vi "MyCircBuffTest.vi"() -> ()   [LabVIEW 2013]
uses:
  My circular buffer info.ctl
panel:
  in  "stop":bool
  in  "Event Click":bool
  out "Waveform Graph":i16[][](graph)
  out "write pointer (block position)":i32
  in  "buffer2 path":path
  in  "buffer1 path":path
  in  "archive directory":path
  in  "num blocks  prior":i32
  in  "num blocks after":i32
  in  "bytes/sample":i32
  in  "samples/block/channel":i32
  in  "number of channels":i32
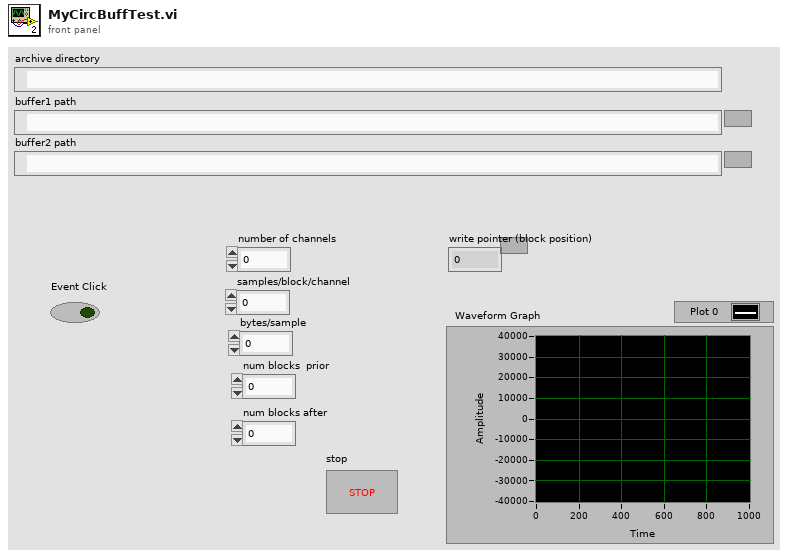
[diagram p1: front panel]
types:
  T1 = typedef "My circular buffer info.ctl" = cluster{"buff ref1":refnum<file>, "buff ref2":refnum<file>, "buffer1 path":path, "buffer2 path":path, "archive directory":path, "xml header":string, "num blocks  prior":i32, "num blocks after":i32, "blocks/event":i32, "samples/block":i32, "bytes/sample":i32, "number of channels":i32, "samples/block/channel":i32, "read buffer ref queue":refnum<queue>, "Event delay queue":refnum<queue>, "command queue":refnum<queue>}
  T2 = cluster{"filename":string, "bytes to write":i32, "archive mode":enum16{"direct", "append"}}
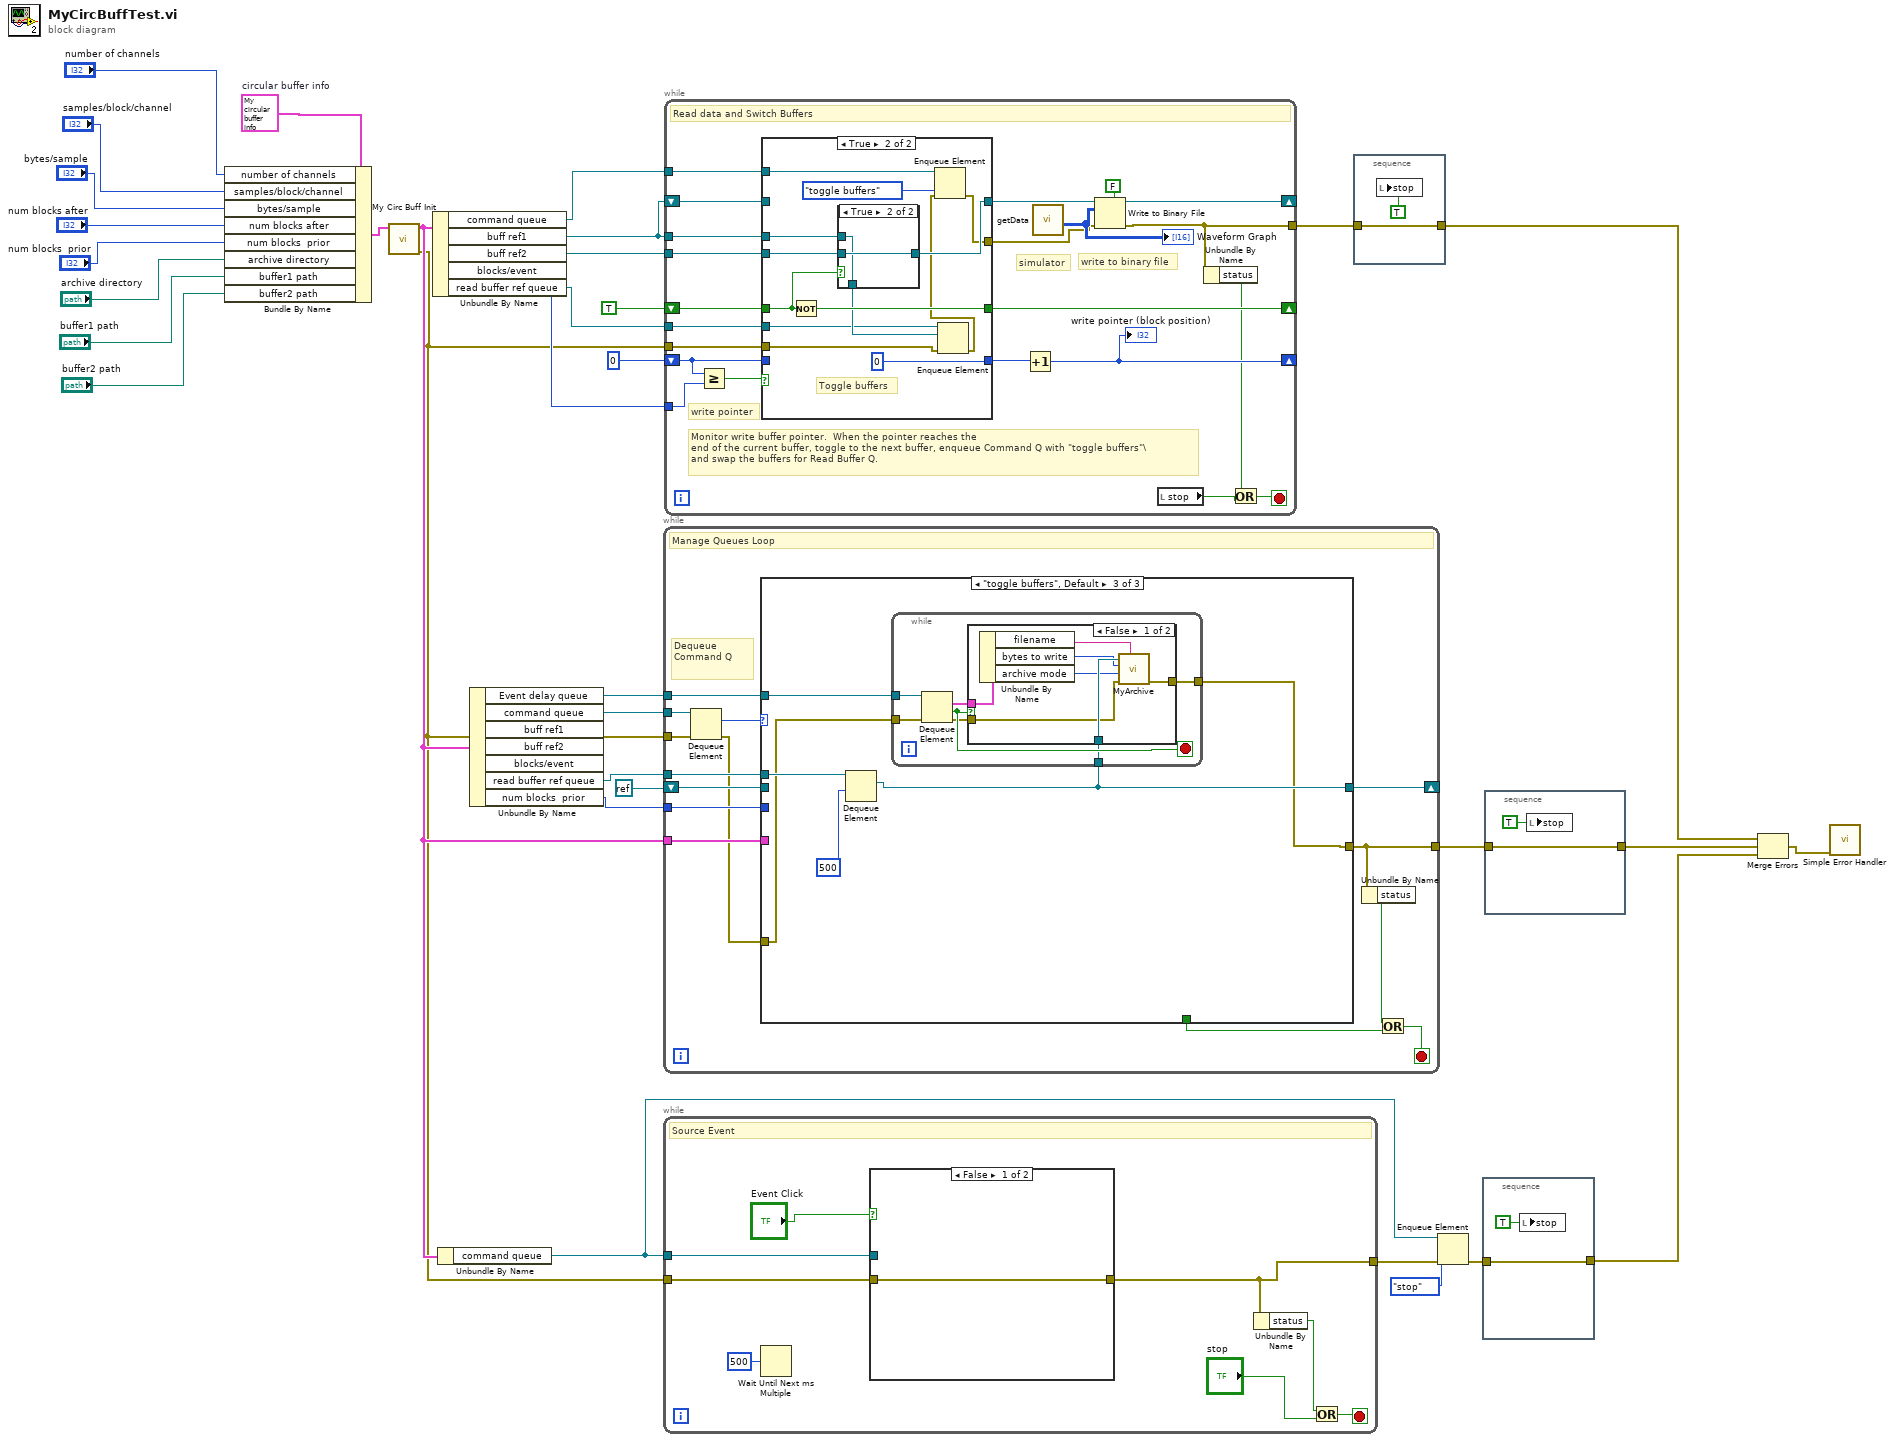
[diagram p0: block diagram]
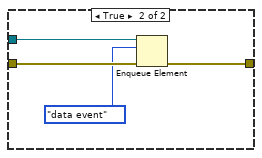
[diagram p2: hidden frame]
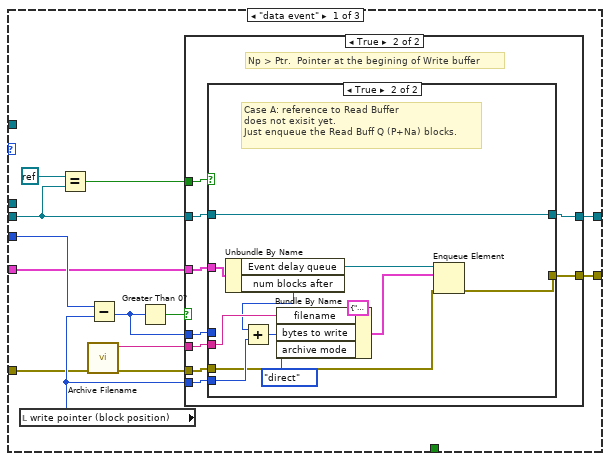
[diagram p3: hidden frame]
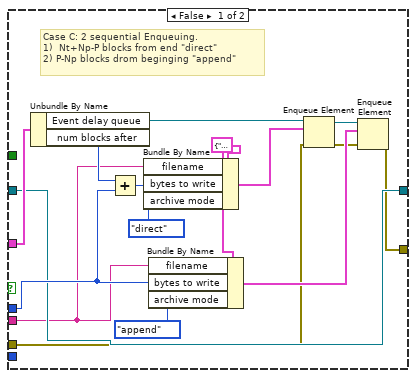
[diagram p4: hidden frame]
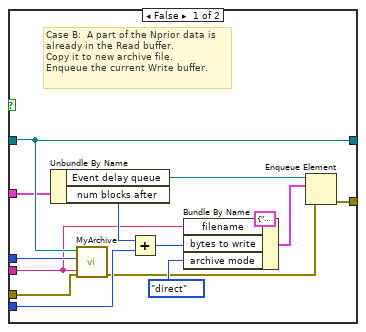
[diagram p5: hidden frame]
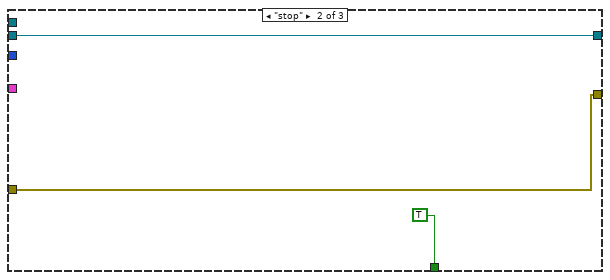
[diagram p6: hidden frame]
diagram:
  w29 = T1 {"buff ref1"=refnum, "buff ref2"=refnum, "buffer1 path"=path "", "buffer2 path"=path "", "archive directory"=path "", "xml header"="", "num blocks  prior"=0, "num blocks after"=0, "blocks/event"=0, "samples/block"=0, "bytes/sample"=0, "number of channels"=0, "samples/block/channel"=0, "read buffer ref queue"=refnum, "Event delay queue"=refnum, "command queue"=refnum}  # circular buffer info
  n1 = Bundle By Name(cluster=w29, "number of channels"="number of channels", "samples/block/channel"="samples/block/channel", "bytes/sample"="bytes/sample", "num blocks after"="num blocks after", "num blocks  prior"="num blocks  prior", "archive directory"="archive directory", "buffer1 path"="buffer1 path", "buffer2 path"="buffer2 path") -> (w25:T1)
  n2 = call "My Circ Buff Init.vi"("circular buffer info"=w25) -> ("error out"=w6:errorcluster, "circular buffer info out"=w12:T1)  [unwired: 9 in]
  n3 = Unbundle By Name(w12) -> ("command queue"=w18:refnum<queue>, "buff ref1"=w20:refnum<file>, "buff ref2"=w22:refnum<file>, "blocks/event"=w24:i32, "read buffer ref queue"=w19:refnum<queue>)
  n4 = Unbundle By Name(w12) -> ("command queue"=w11:refnum<queue>)
  n5 = Unbundle By Name(w12) -> ("Event delay queue"=w13:refnum<queue>, "command queue"=w17:refnum<queue>, "read buffer ref queue"=w14:refnum<queue>, "num blocks  prior"=w15:i32)  [unwired: 3 out]
  n6 = while {
    tunnel: w17 -> [w48]
    shift-right: [w44] -> _
    shift-left: refnum<k0> refnum -> [w47]
    tunnel: w15 -> [w46]
    tunnel: w12 -> [w45]
    tunnel: w14 -> [w43]
    tunnel: w13 -> [w42]
    tunnel: w6 -> [w41]
    tunnel: [w39] -> w7
    stop <- w36 stop-if-true
    # "Dequeue \nCommand Q"
    # "Manage Queues Loop"
    n7 = Dequeue Element(queue=w48, error in (no error)=w41) -> (element=w35:enum16{"toggle buffers", "data event", "stop"}, error out=w40:errorcluster)  [unwired: 1 in, 2 out]
    n8 = case shown="\"toggle buffers\", Default" w35 {
      tunnel: w47 -> [w55 w115 _]
      tunnel: w46 -> [w59 _ _]
      tunnel: w45 -> [w57 _ _]
      tunnel: [w54 w115 w119] -> w44
      tunnel: w43 -> [_ _ w121]
      tunnel: w42 -> [_ _ w120]
      tunnel: [_ TRUE _] -> w37
      tunnel: w40 -> [w51 w113 w117]
      tunnel: [w49 w113 w116] -> w39
      frame "data event" {
        n9 = local read "write pointer (block position)"() -> (w52:i32)
        n10 = Equal?(x=refnum<k0> refnum, y=w55) -> (x = y?=w60:bool)
        n11 = call "Archive Filename.vi"("error in (no error)"=w51) -> ("error out"=w50:errorcluster, "filename"=w53:string)  [unwired: 9 in]
        n12 = Subtract(x=w59, y=w52) -> (x-y=w56:i32)
        n13 = Greater Than 0?(x=w56) -> (x > 0?=w58:bool)
        n14 = case shown="True" w58 {
          tunnel: w60 -> [_ w86]
          tunnel: w57 -> [w67 w85]
          tunnel: w56 -> [w70 w84]
          tunnel: w55 -> [w66 w83]
          tunnel: [w66 w82] -> w54
          tunnel: w53 -> [w65 w81]
          tunnel: w52 -> [_ w80]
          tunnel: w50 -> [w64 w79]
          tunnel: [w62 w78] -> w49
          frame False {
            w69 = T2 {"filename"="", "bytes to write"=0, "archive mode"=enum."direct"} ("Event delay info")
            # "Case C: 2 sequential Enqueuing. \n1)  Nt+Np-P blocks from end \"direct\"\n2) P-Np blocks drom beginging \"append\""
            n15 = Unbundle By Name(w67) -> ("Event delay queue"=w77:refnum<queue>, "num blocks after"=w73:i32)
            n16 = Add(x=w73, y=w70) -> (x+y=w74:i32)
            n17 = Bundle By Name(cluster=w69, "filename"=w65, "bytes to write"=w74, "archive mode"=enum16{"direct", "append"}."direct") -> (w75:T2)
            n18 = Bundle By Name(cluster=w69, "filename"=w65, "bytes to write"=w70, "archive mode"=enum16{"direct", "append"}."append") -> (w68:T2)
            n19 = Enqueue Element(queue=w77, element=w75, error in (no error)=w64) -> (queue out=w72:refnum<queue>, error out=w63:errorcluster)  [unwired: 1 in, 1 out]
            n20 = Enqueue Element(queue=w72, element=w68, error in (no error)=w63) -> (error out=w62:errorcluster)  [unwired: 1 in, 2 out]
          }
          frame True {
            # "Np > Ptr.  Pointer at the begining of Write buffer"
            n21 = case shown="True" w86 {
              tunnel: w85 -> [w93 w112]
              tunnel: w84 -> [w100 _]
              tunnel: w83 -> [w99 w107]
              tunnel: [w99 w107] -> w82
              tunnel: w81 -> [w90 w106]
              tunnel: w80 -> [w92 w103]
              tunnel: w79 -> [w89 w102]
              tunnel: [w87 w101] -> w78
              frame False {
                # "Case B:  A part of the Nprior data is\nalready in the Read buffer.  \nCopy it to new archive file.\nEnqueue the current Write buffer."
                n22 = Unbundle By Name(w93) -> ("Event delay queue"=w98:refnum<queue>, "num blocks after"=w91:i32)
                n23 = call "MyArchive.vi"("archive filename"=w90, "error in"=w89, "blocks to write"=w100, "ReadBuff refnum"=w99) -> ("error out"=w88:errorcluster)  [unwired: 5 in]
                n24 = Add(x=w91, y=w92) -> (x+y=w94:i32)
                n25 = Bundle By Name(cluster=T2 {"filename"="", "bytes to write"=0, "archive mode"=enum."direct"} ("Event delay info"), "filename"=w90, "bytes to write"=w94, "archive mode"=enum16{"direct", "append"}."direct") -> (w95:T2)
                n26 = Enqueue Element(queue=w98, element=w95, error in (no error)=w88) -> (error out=w87:errorcluster)  [unwired: 1 in, 2 out]
              }
              frame True {
                # "Case A: reference to Read Buffer \ndoes not exisit yet. \nJust enqueue the Read Buff Q (P+Na) blocks."
                n27 = Unbundle By Name(w112) -> ("Event delay queue"=w111:refnum<queue>, "num blocks after"=w104:i32)
                n28 = Add(x=w104, y=w103) -> (x+y=w105:i32)
                n29 = Bundle By Name(cluster=T2 {"filename"="", "bytes to write"=0, "archive mode"=enum."direct"} ("Event delay info"), "filename"=w106, "bytes to write"=w105, "archive mode"=enum16{"direct", "append"}."direct") -> (w108:T2)
                n30 = Enqueue Element(queue=w111, element=w108, error in (no error)=w102) -> (error out=w101:errorcluster)  [unwired: 1 in, 2 out]
              }
            }
          }
        }
      }
      frame "stop" {
      }
      frame "toggle buffers", Default {
        n31 = Dequeue Element(queue=w121, timeout in ms (-1)=500) -> (element=w119:refnum<file>)  [unwired: 1 in, 3 out]
        n32 = while {
          tunnel: w120 -> [w128]
          tunnel: w119 -> [w126]
          tunnel: w117 -> [w124]
          tunnel: [w122] -> w116
          stop <- w127 stop-if-true
          n33 = Dequeue Element(queue=w128, error in (no error)=w124) -> (element=w125:T2, timed out?=w127:bool, error out=w123:errorcluster)  [unwired: 1 in, 1 out]
          n34 = case shown="False" w127 {
            tunnel: w126 -> [w135 _]
            tunnel: w125 -> [w134 _]
            tunnel: w123 -> [w130 w136]
            tunnel: [w129 w136] -> w122
            frame False {
              n35 = Unbundle By Name(w134) -> ("filename"=w131:string, "bytes to write"=w132:i32, "archive mode"=w133:enum16{"direct", "append"})
              n36 = call "MyArchive.vi"("archive filename"=w131, "error in"=w130, "archive mode"=w133, "blocks to write"=w132, "ReadBuff refnum"=w135) -> ("error out"=w129:errorcluster)  [unwired: 4 in]
            }
            frame True {
              # "no event waits"
            }
          }
        }
      }
    }
    n37 = Unbundle By Name(w39) -> ("status"=w38:bool)
    n38 = Or(x=w38, y=w37) -> (x .or. y?=w36:bool)
  }
  n39 = while {
    tunnel: w11 -> [w144]
    tunnel: w6 -> [w143]
    tunnel: [w141] -> w5
    stop <- w142 stop-if-true
    # "Source Event"
    n40 = Wait Until Next ms Multiple(millisecond multiple=u32 500) -> ()  [unwired: 1 out]
    n41 = case shown="False" "Event Click" {
      tunnel: w144 -> [_ w149]
      tunnel: w143 -> [w145 w148]
      tunnel: [w145 w147] -> w141
      frame False {
      }
      frame True {
        n42 = Enqueue Element(queue=w149, element=enum16{"data event", "toggle buffers", "stop"}."data event", error in (no error)=w148) -> (error out=w147:errorcluster)  [unwired: 1 in, 2 out]
      }
    }
    n43 = Unbundle By Name(w141) -> ("status"=w140:bool)
    n44 = Or(x=w140, y="stop") -> (x .or. y?=w142:bool)
  }
  n45 = while {
    tunnel: w24 -> [w170]
    shift-right: [w166] -> _
    shift-left: 0 -> [w168]
    shift-right: [w163] -> _
    shift-left: w20 -> [w164]
    tunnel: w22 -> [w162]
    shift-right: [w160] -> _
    shift-left: TRUE -> [w161]
    tunnel: w20 -> [w159]
    tunnel: w19 -> [w158]
    tunnel: w18 -> [w157]
    tunnel: w6 -> [w155]
    tunnel: [w151] -> w8
    stop <- w153 stop-if-true
    # "Monitor write buffer pointer.  When the pointer reaches the \nend of the current buffer, toggle to the next buffer, enqueue Command Q with \"toggle buffers\"\\\nand swap the buffers for Read Buffer Q."
    # "write pointer"
    # "simulator"
    # "write to binary file"
    # "Read data and Switch Buffers"
    n46 = Greater Or Equal?(x=w168, y=w170) -> (x >= y?=w169:bool)
    n47 = case shown="True" w169 {
      tunnel: w168 -> [w175 _]
      tunnel: [w175 0] -> w167
      tunnel: [w174 w185] -> w165
      tunnel: w164 -> [w174 _]
      tunnel: w162 -> [_ w186]
      tunnel: w161 -> [w173 w187]
      tunnel: [w173 w188] -> w160
      tunnel: w159 -> [_ w184]
      tunnel: w158 -> [_ w182]
      tunnel: w157 -> [_ w181]
      tunnel: w155 -> [w172 w179]
      tunnel: [w172 w177] -> w154
      frame False {
      }
      frame True {
        # "Toggle buffers"
        n48 = Not(x=w187) -> (.not. x?=w188:bool)
        n49 = case shown="True" w187 {
          tunnel: w186 -> [w189 w192]
          tunnel: [w190 w192] -> w185
          tunnel: w184 -> [w190 w191]
          tunnel: [w189 w191] -> w183
          frame False {
          }
          frame True {
          }
        }
        n50 = Enqueue Element(queue=w182, element=w183, error in (no error)=w179) -> (error out=w178:errorcluster)  [unwired: 1 in, 2 out]
        n51 = Enqueue Element(queue=w181, element=enum16{"toggle buffers", "data event", "stop"}."toggle buffers", error in (no error)=w178) -> (error out=w177:errorcluster)  [unwired: 1 in, 2 out]
      }
    }
    n52 = Increment(x=w167) -> (x+1=w166:i32)
    "write pointer (block position)" <- w166
    n53 = call "getData.vi"() -> ("binary data"=w156:i16[][])  [unwired: 7 in]
    "Waveform Graph" <- w156
    n54 = Write to Binary File(file (use dialog)=w165, data=w156, error in=w154, 5:FALSE ("prepend array or string size? (T)")) -> (refnum out=w163:refnum<file>, error out=w151:errorcluster)  [unwired: 2 in, 1 out]
    n55 = local read "stop"() -> (w152:bool)
    n56 = Unbundle By Name(w151) -> ("status"=w150:bool)
    n57 = Or(x=w150, y=w152) -> (x .or. y?=w153:bool)
  }
  n58 = stacked-sequence {
    tunnel: w8 -> [w194]
    tunnel: [w194] -> w4
    frame #0 {
      n59 = local write "stop"(TRUE ("stop")) -> ()
    }
  }
  n60 = Enqueue Element(queue=w11, element=enum16{"data event", "toggle buffers", "stop"}."stop", error in (no error)=w5) -> (error out=w9:errorcluster)  [unwired: 1 in, 2 out]
  n61 = stacked-sequence {
    tunnel: w9 -> [w196]
    tunnel: [w196] -> w2
    frame #0 {
      n62 = local write "stop"(TRUE ("stop")) -> ()
    }
  }
  n63 = stacked-sequence {
    tunnel: w7 -> [w198]
    tunnel: [w198] -> w3
    frame #0 {
      n64 = local write "stop"(TRUE ("stop")) -> ()
    }
  }
  n65 = Merge Errors(w4, w3, w2) -> (w1:errorcluster)
  n66 = call <vilib>:"Simple Error Handler.vi"("error in (no error)"=w1) -> ()  [unwired: 4 in, 5 out]
